vi "bcd_too_7seg_decoder.vi"(0 "A":bool, 5 "B":bool, 7 "C":bool, 9 "D":bool) -> (3 "?":bool, 4 "?":bool, 6 "?":bool, 8 "?":bool, 10 "?":bool, 14 "?":bool, 15 "?":bool)   [LabVIEW 2015]
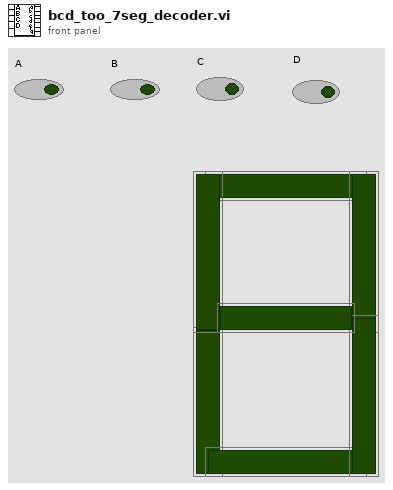
[diagram p1: front panel]
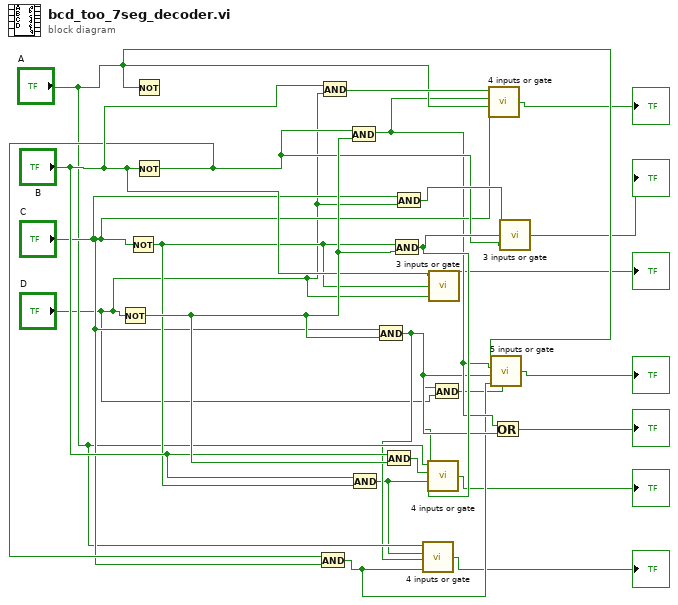
[diagram p0: block diagram]
diagram:
  n1 = Not(x="D") -> (.not. x?=w21:bool)
  n2 = Not(x="C") -> (.not. x?=w19:bool)
  n3 = Not(x="A") -> ()  [unwired: 1 out]
  n4 = Not(x="B") -> (.not. x?=w16:bool)
  n5 = And(x=w16, y="C") -> (x .and. y?=w11:bool)
  n6 = And(x="B", y="D") -> (x .and. y?=w23:bool)
  n7 = And(x=w16, y=w21) -> (x .and. y?=w13:bool)
  n8 = And(x="B", y=w19) -> (x .and. y?=w8:bool)
  n9 = And(x="C", y=w21) -> (x .and. y?=w12:bool)
  n10 = And(x="B", y=w21) -> (x .and. y?=w18:bool)
  n11 = And(x=w19, y=w21) -> (x .and. y?=w17:bool)
  n12 = And(x="C", y="D") -> (x .and. y?=w22:bool)
  n13 = call "4 inputs or gate.vi"("p"=w11, "z"=w12, "y"=w8, "x"="A") -> ("o2"=→"?":bool)
  n14 = call "4 inputs or gate.vi"("p"=w17, "z"=w8, "y"=w18, "x"="A") -> ("o2"=→"?":bool)
  n15 = call "3 inputs or gate.vi"("z"="D", "y"=w19, "x"="B") -> ("o1"=→"?":bool)
  n16 = And(x=w8, y="D") -> (x .and. y?=w10:bool)
  n17 = call "4 inputs or gate.vi"("p"="C", "z"="A", "y"=w13, "x"=w23) -> ("o2"=→"?":bool)
  n18 = call "5 inputs or gate.vi"("x"="A", "y"=w13, "z"=w12, "p"=w11, "m"=w10) -> ("o3"=→"?":bool)
  n19 = Or(x=w13, y=w12) -> (x .or. y?=→"?":bool)
  n20 = call "3 inputs or gate.vi"("z"=w16, "y"=w17, "x"=w22) -> ("o1"=→"?":bool)
